vi "Write Center Point.vi"(10 "Center Point":dbl[unit], 11 "PressureServoCylinderActuator in":refnum<class "FlowControlActuator.lvclass">) -> (3 "PressureServoCylinderActuator out":refnum<class "FlowControlActuator.lvclass">)   [LabVIEW 2015, in "FlowControlActuator.lvclass"]
uses:
  FlowControlActuator.lvclass
  FlowControlActuator.lvclass/FlowControlActuator.ctl
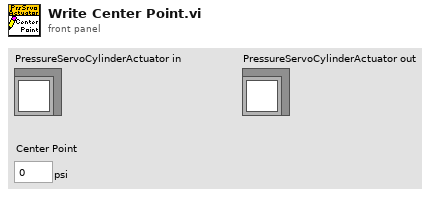
[diagram p1: front panel]
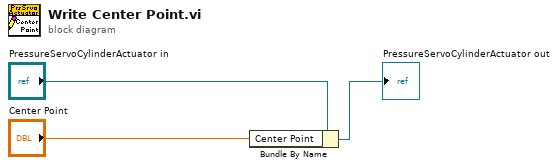
[diagram p0: block diagram]
diagram:
  n1 = Bundle By Name(cluster="PressureServoCylinderActuator in", "Center Point"="Center Point") -> (→"PressureServoCylinderActuator out":refnum<class "FlowControlActuator.lvclass">)
